vi "Exercise 3-9.vi"(6 "Max Wind Speed":dbl, 7 "Current Wind Speed":dbl, 9 "Min Temp":dbl, 10 "Max Temp":dbl, 11 "Current Temp":dbl) -> (1 "Warning?":bool, 2 "Warning Text":string)   [LabVIEW 2014]
doc: "This VI is an exercise in the LabVIEW Core I course. In this exercise, you generate appropriate strings for Freeze, Heat Stroke, and High Wind warnings, and combinations of the warnings."
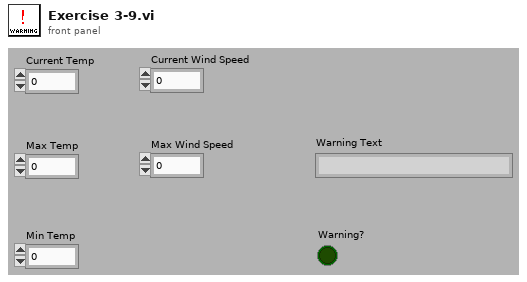
[diagram p1: front panel]
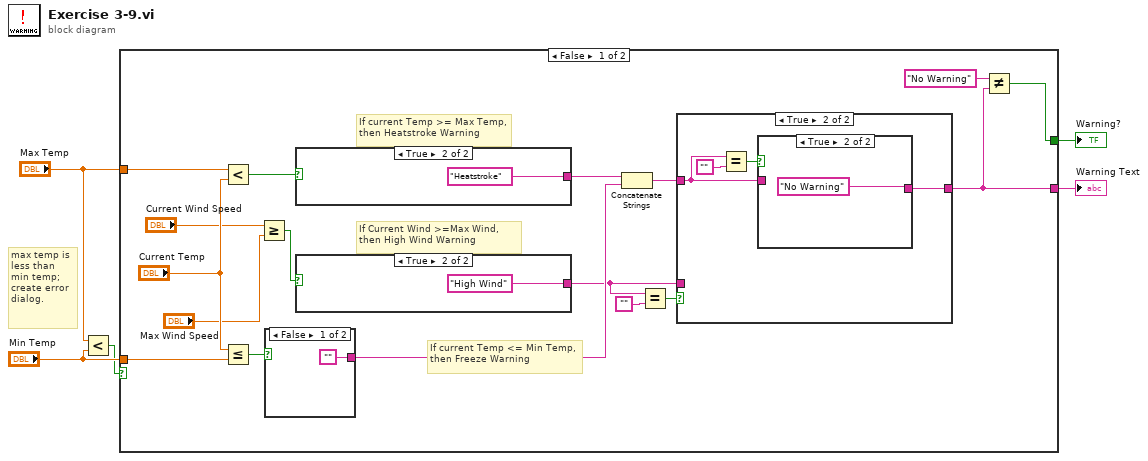
[diagram p0: block diagram]
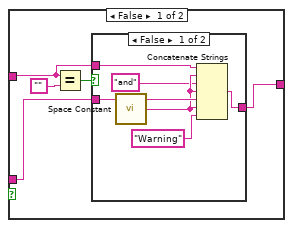
[diagram p2: hidden frame]
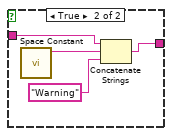
[diagram p3: hidden frame]
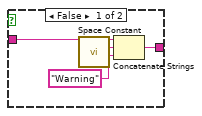
[diagram p4: hidden frame]
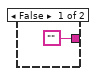
[diagram p5: hidden frame]
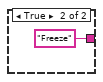
[diagram p6: hidden frame]
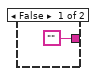
[diagram p7: hidden frame]
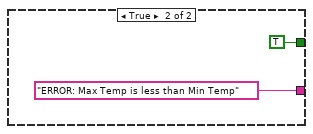
[diagram p8: hidden frame]
diagram:
  # "max temp is less than min temp; create error dialog."
  n1 = Less?(x="Max Temp", y="Min Temp") -> (x < y?=w1:bool)
  n2 = case shown="False" w1 {
    tunnel: [w6 TRUE] -> w5
    tunnel: [w8 "ERROR: Max Temp is less than Min Temp"] -> w4
    tunnel: "Max Temp" -> [w16 _]
    tunnel: "Min Temp" -> [w15 _]
    frame False {
      # "If Current Wind >=Max Wind, then High Wind Warning"
      # "If current Temp <= Min Temp, then Freeze Warning"
      # "If current Temp >= Max Temp, then Heatstroke Warning"
      n3 = Less?(x=w16, y="Current Temp") -> (x < y?=w20:bool)
      n4 = Less Or Equal?(x="Current Temp", y=w15) -> (x <= y?=w22:bool)
      n5 = Greater Or Equal?(x="Current Wind Speed", y="Max Wind Speed") -> (x >= y?=w17:bool)
      n6 = case shown="False" w22 {
        tunnel: ["" "Freeze"] -> w13
        frame False {
        }
        frame True {
        }
      }
      n7 = case shown="True" w20 {
        tunnel: ["" "Heatstroke"] -> w14
        frame False {
        }
        frame True {
        }
      }
      n8 = case shown="True" w17 {
        tunnel: ["" "High Wind"] -> w9
        frame False {
        }
        frame True {
        }
      }
      n9 = Concatenate Strings(w14, w13) -> (w10:string)
      n10 = Equal?(x=w9, y="") -> (x = y?=w11:bool)
      n11 = case shown="True" w11 {
        tunnel: w10 -> [w24 w39]
        tunnel: w9 -> [w25 _]
        tunnel: [w23 w38] -> w8
        frame False {
          n12 = Equal?(x=w24, y="") -> (x = y?=w27:bool)
          n13 = case shown="False" w27 {
            tunnel: w25 -> [w33 w35]
            tunnel: [w31 w36] -> w23
            tunnel: w24 -> [w30 _]
            frame False {
              n14 = call <vilib>:"Space Constant.vi"() -> ("String"=w29:string)
              n15 = Concatenate Strings(w30, w29, "and", w29, w33, w29, "Warning") -> (w31:string)
            }
            frame True {
              n16 = call <vilib>:"Space Constant.vi"() -> ("String"=w34:string)
              n17 = Concatenate Strings(w35, w34, "Warning") -> (w36:string)
            }
          }
        }
        frame True {
          n18 = Equal?(x=w39, y="") -> (x = y?=w41:bool)
          n19 = case shown="True" w41 {
            tunnel: w39 -> [w45 _]
            tunnel: [w42 "No Warning"] -> w38
            frame False {
              n20 = call <vilib>:"Space Constant.vi"() -> ("String"=w44:string)
              n21 = Concatenate Strings(w45, w44, "Warning") -> (w42:string)
            }
            frame True {
            }
          }
        }
      }
      n22 = Not Equal?(x="No Warning", y=w8) -> (x != y?=w6:bool)
    }
    frame True {
    }
  }
  "Warning Text" <- w4
  "Warning?" <- w5
